vi "Get Range.vi"(7 "Ref Range":refnum<vi>, 8 "error in":errorcluster, 9 "Head Channel":i16, 10 "Pulsar Handle":i16, 11 "OphirFastX (in)":refnum<k7>) -> (0 "error out":errorcluster, 3 "OphirFastX (out)":refnum<k7>)   [LabVIEW 2009]
panel:
  # "Guillaume Plateau - yguig2@yahoo.fr"
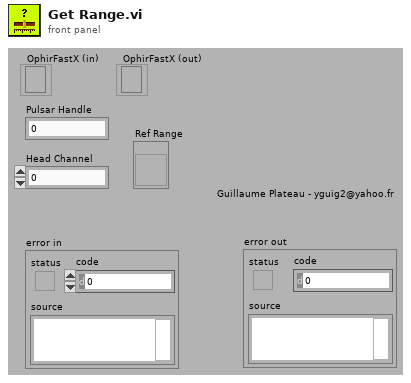
[diagram p1: front panel]
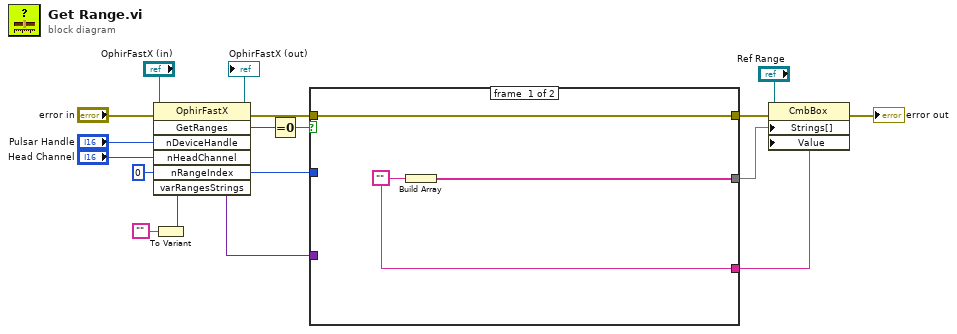
[diagram p0: block diagram]
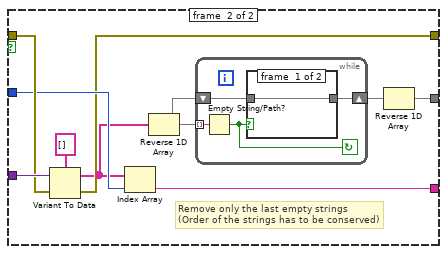
[diagram p2: hidden frame]
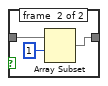
[diagram p3: hidden frame]
diagram:
  n1 = To Variant(anything="") -> (Variant=w11:variant)
  n2 = invoke class="OphirFastX" method="GetRanges"(reference="OphirFastX (in)", error in="error in", "nDeviceHandle"="Pulsar Handle", "nHeadChannel"="Head Channel", "nRangeIndex"=i16 0, "varRangesStrings"=w11) -> (reference out=→"OphirFastX (out)":refnum<k7>, error out=w14:errorcluster, "GetRanges"=w12:i32, "nRangeIndex"=w15:i16, "varRangesStrings"=w16:variant)  [unwired: 1 in, 2 out]
  n3 = Equal To 0?(x=w12) -> (x = 0?=w13:bool)
  n4 = case shown="True" w13 {
    tunnel: w16 -> [_ w31]
    tunnel: w14 -> [w20 w30]
    tunnel: w15 -> [_ w28]
    tunnel: [w21 w27] -> w3
    tunnel: [w20 w26] -> w5
    tunnel: [w19 w22] -> w1
    frame #0 {
      w21 = ""
      n5 = Build Array(w21) -> (w19:string[])
    }
    frame #1 {
      # "Remove only the last empty strings\n(Order of the strings has to be conserved)"
      n6 = Variant To Data(error in=w30, Variant=w31, type=string[] []) -> (error out=w26:errorcluster, data=w23:string[])
      n7 = Index Array(array=w23, index=w28) -> (element=w27:string)
      n8 = Reverse 1D Array(array=w23) -> (reversed array=w25:string[])
      n9 = while {
        tunnel: w25 -> [w35] mode=indexing
        shift-right: [w33] -> w24
        shift-left: w25 -> [w34]
        stop <- w32 continue-if-true
        n10 = Empty String/Path?(string/path=w35) -> (empty?=w32:bool)
        n11 = case shown="True" w32 {
          tunnel: w34 -> [w36 w39]
          tunnel: [w36 w37] -> w33
          frame #0 {
          }
          frame #1 {
            n12 = Array Subset(array=w39, index=1) -> (w37:string[])  [unwired: 1 in]
          }
        }
      }
      n13 = Reverse 1D Array(array=w24) -> (reversed array=w22:string[])
    }
  }
  n14 = property class="CmbBox"(reference="Ref Range", error in=w5, "Strings[]"=w1, "Value"=w3) -> (error out=→"error out":errorcluster)  [unwired: 1 out]
